vi "System Definition Control Addon API.vi"() -> ()   [LabVIEW 2013]
uses:
  Shared/Types/Controller Settings.ctl
  Shared/Types/PID Parameters.ctl
  Shared/Types/Industrial Parameters.ctl
  NationalInstruments.VeriStand.SystemDefinitionAPI
  System Definition API/Control SysDef API.lvlib
  Shared/Control Addon Shared.lvlib
panel:
  in  "error in (no error)":errorcluster
  out "Sysdef Path":path=path "C:/Users/Public/Documents/National Instruments/NI VeriStand 2011/Projects/DynamicallyCreatedProject/DynamicallyCreatedProject.nivssdf"
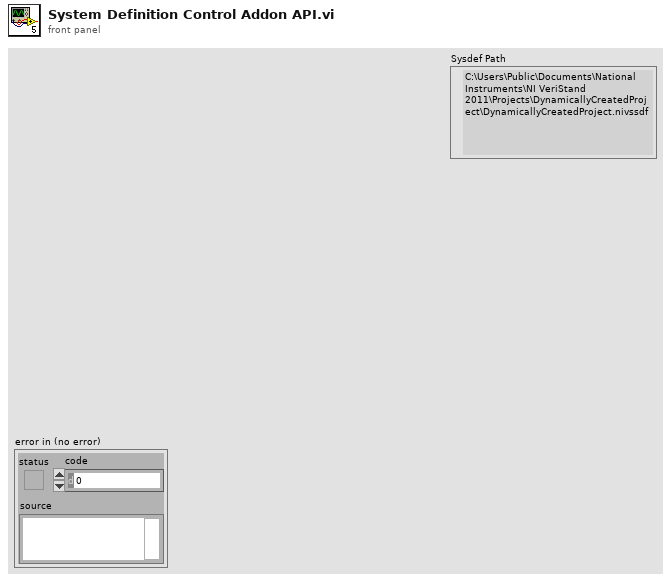
[diagram p1: front panel]
types:
  T1 = typedef "Control Addon Shared.lvlib/Controller Settings.ctl" = cluster{"Output Max":dbl, "Output Min":dbl, "Setpoint Max":dbl, "Setpoint Min":dbl, "Use External Setpoint":bool, "Output Rate Limiter":dbl}
  T2 = typedef "Control Addon Shared.lvlib/Industrial Parameters.ctl" = cluster{"Enable Hysteresis":bool, "Hysteresis":dbl, "Enable Filter":bool, "Minimum Switching":dbl}
  T3 = cluster{"Channel Linkages":cluster{"Feedback Node Path":string, "Output Node Path":string, "Setpoint Node Path":string}, "Controller Settings":T1, "Parameters":T2, "Name":string}
  T4 = typedef "Control Addon Shared.lvlib/PID Parameters.ctl" = cluster{"Enable Live Updates":bool, "Enable Gain Scheduling":bool, "PID Parameters":dbl[][]}
  T5 = cluster{"Channel Linkages":cluster{"Feedback Node Path":string, "Output Node Path":string, "Setpoint Node Path":string, "Gain Schedule Node Path":string}, "Controller Settings":T1, "Parameters":T4, "Name":string}
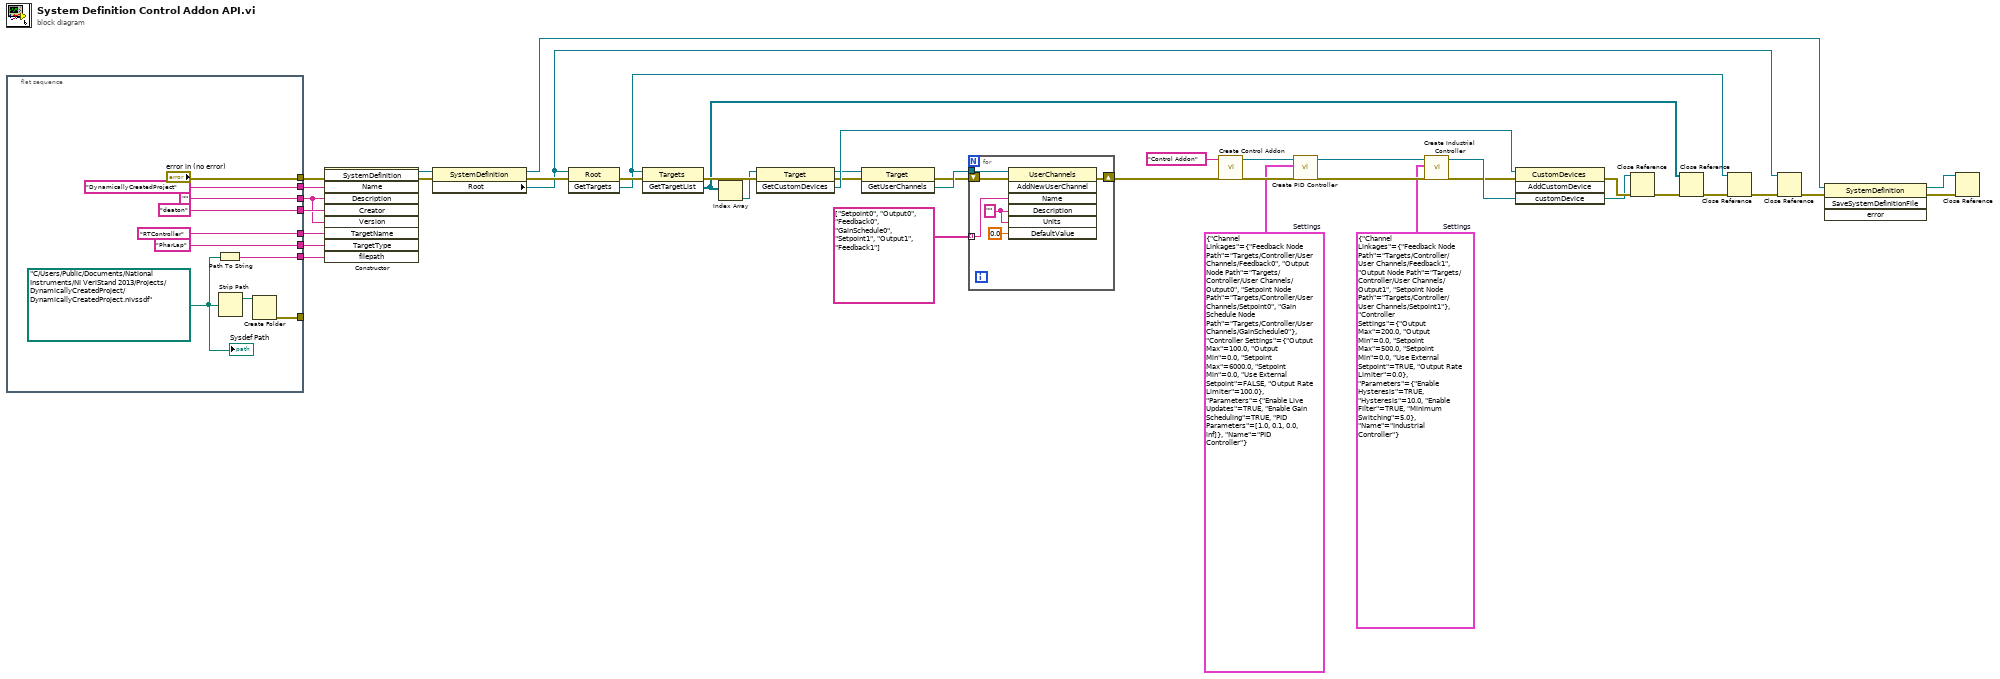
[diagram p0: block diagram]
diagram:
  w7 = T3 {"Channel Linkages"={"Feedback Node Path"="Targets/Controller/User Channels/Feedback1", "Output Node Path"="Targets/Controller/User Channels/Output1", "Setpoint Node Path"="Targets/Controller/User Channels/Setpoint1"}, "Controller Settings"={"Output Max"=200.0, "Output Min"=0.0, "Setpoint Max"=500.0, "Setpoint Min"=0.0, "Use External Setpoint"=TRUE, "Output Rate Limiter"=0.0}, "Parameters"={"Enable Hysteresis"=TRUE, "Hysteresis"=10.0, "Enable Filter"=TRUE, "Minimum Switching"=5.0}, "Name"="Industrial Controller"}  # Settings
  w8 = T5 {"Channel Linkages"={"Feedback Node Path"="Targets/Controller/User Channels/Feedback0", "Output Node Path"="Targets/Controller/User Channels/Output0", "Setpoint Node Path"="Targets/Controller/User Channels/Setpoint0", "Gain Schedule Node Path"="Targets/Controller/User Channels/GainSchedule0"}, "Controller Settings"={"Output Max"=100.0, "Output Min"=0.0, "Setpoint Max"=6000.0, "Setpoint Min"=0.0, "Use External Setpoint"=FALSE, "Output Rate Limiter"=100.0}, "Parameters"={"Enable Live Updates"=TRUE, "Enable Gain Scheduling"=TRUE, "PID Parameters"=[[1.0, 0.1, 0.0, inf]]}, "Name"="PID Controller"}  # Settings
  n1 = flat-sequence {
    tunnel: ["DynamicallyCreatedProject" ("Name")] -> w38
    tunnel: ["deaton" ("Creator")] -> w37
    tunnel: ["RTController" ("TargetName")] -> w26
    tunnel: ["PharLap" ("TargetType")] -> w36
    tunnel: ["" ("Description")] -> w35
    tunnel: [w43] -> w34
    tunnel: [w42] -> _
    tunnel: ["error in (no error)"] -> w27
    frame #0 {
      w44 = path "C:/Users/Public/Documents/National Instruments/NI VeriStand 2013/Projects/DynamicallyCreatedProject/DynamicallyCreatedProject.nivssdf"
      n2 = Path To String(path=w44) -> (string=w43:string)
      n3 = Strip Path(path=w44) -> (stripped path=w45:path)  [unwired: 1 out]
      n4 = Create Folder(path (use dialog)=w45) -> (error out=w42:errorcluster)  [unwired: 2 in, 2 out]
      "Sysdef Path" <- w44
    }
  }
  n5 = constructor class="SystemDefinition"(error in=w27, "Name"=w38, "Description"=w35, "Creator"=w37, "Version"=w35, "TargetName"=w26, "TargetType"=w36, "filepath"=w34) -> (reference out=w31:refnum<k24>, error out=w33:errorcluster)  [unwired: 2 in, 8 out]
  n6 = property class="SystemDefinition"(reference=w31, error in=w33) -> (reference out=w11:refnum<k24>, error out=w32:errorcluster, "Root"=w12:refnum<k24>)
  n7 = invoke class="Root" method="GetTargets"(reference=w12, error in=w32) -> (error out=w30:errorcluster, "GetTargets"=w14:refnum<k24>)  [unwired: 1 in, 1 out]
  n8 = invoke class="Targets" method="GetTargetList"(reference=w14, error in=w30) -> (error out=w25:errorcluster, "GetTargetList"=w16:refnum<k24>[])  [unwired: 1 in, 1 out]
  n9 = Index Array(array=w16) -> (element=w24:refnum<k24>)  [unwired: 1 in]
  n10 = invoke class="Target" method="GetCustomDevices"(reference=w24, error in=w25) -> (reference out=w6:refnum<k24>, error out=w5:errorcluster, "GetCustomDevices"=w18:refnum<k24>)  [unwired: 1 in]
  n11 = invoke class="Target" method="GetUserChannels"(reference=w6, error in=w5) -> (error out=w3:errorcluster, "GetUserChannels"=w4:refnum<k24>)  [unwired: 1 in, 1 out]
  n12 = for {
    tunnel: w4 -> [w56]
    shift-right: [w54] -> w2
    shift-left: w3 -> [w55]
    tunnel: string[] ["Setpoint0", "Output0", "Feedback0", "GainSchedule0", "Setpoint1", "Output1", "Feedback1"] -> [w53] mode=indexing
    w51 = "" ("Units")
    n13 = invoke class="UserChannels" method="AddNewUserChannel"(reference=w56, error in=w55, "Name"=w53, "Description"=w51, "Units"=w51, "DefaultValue"=0.0) -> (error out=w54:errorcluster)  [unwired: 1 in, 6 out]
  }
  n14 = call "Create Control Addon.vi"("error in (no error)"=w2, "Name"="Control Addon") -> ("error out"=w19:errorcluster, "Custom Device Ref"=w39:refnum<k24>)  [unwired: 8 in]
  n15 = call "Create PID Controller.vi"("error in (no error)"=w19, "Settings"=w8, "Custom Device Ref"=w39) -> ("error out"=w20:errorcluster, "Custom Device Ref"=w40:refnum<k24>)  [unwired: 7 in]
  n16 = call "Create Industrial Controller.vi"("error in (no error)"=w20, "Settings"=w7, "Custom Device Ref"=w40) -> ("error out"=w21:errorcluster, "Custom Device Ref"=w22:refnum<k24>)  [unwired: 7 in]
  n17 = invoke class="CustomDevices" method="AddCustomDevice"(reference=w18, error in=w21, "customDevice"=w22) -> (error out=w23:errorcluster)  [unwired: 1 in, 3 out]
  n18 = Close Reference(reference=w22, error in (no error)=w23) -> (error out=w17:errorcluster)
  n19 = Close Reference(reference=w16, error in (no error)=w17) -> (error out=w15:errorcluster)
  n20 = Close Reference(reference=w14, error in (no error)=w15) -> (error out=w13:errorcluster)
  n21 = Close Reference(reference=w12, error in (no error)=w13) -> (error out=w10:errorcluster)
  n22 = invoke class="SystemDefinition" method="SaveSystemDefinitionFile"(reference=w11, error in=w10) -> (reference out=w28:refnum<k24>, error out=w29:errorcluster)  [unwired: 2 in, 2 out]
  n23 = Close Reference(reference=w28, error in (no error)=w29) -> ()  [unwired: 1 out]
